vi "test_Set-Get Protocol UDP.vi"(8 "error in (no error)":errorcluster, 11 "TestCase in":refnum<class "Instrument Addon Scripting API Custom Device Unit Tests.lvclass">) -> (0 "error out":errorcluster, 3 "TestCase out":refnum<class "Instrument Addon Scripting API Custom Device Unit Tests.lvclass">)   [LabVIEW 2019, in "Instrument Addon Scripting API Custom Device Unit Tests.lvclass"]
uses:
  Instrument Addon Scripting API Custom Device Unit Tests.lvclass
  Includes/Protocols.lvlibp/UDP/UDP.lvclass
  C:/Users/nitest/Desktop/Git/niveristand-instrument-addon-custom-device/Includes/Protocols.lvlibp/Protocol Parent/Protocol Parent.lvclass
  Includes/Protocols.lvlibp/AK RS-xxx/AK RS-xxx.lvclass
  Instrument Addon Scripting API Custom Device Unit Tests.lvclass/Instrument Addon Scripting API Custom Device Unit Tests.ctl
  Includes/Protocols.lvlibp/UDP/Data Access/Write Local IP Address.vi
  Includes/Protocols.lvlibp/UDP/Data Access/Write Local Port.vi
  Includes/Protocols.lvlibp/UDP/Data Access/Write Target IP Address.vi
  Includes/Protocols.lvlibp/UDP/Data Access/Write Target Port.vi
  Instrument Addon Scripting API Test Assets/Instrument Addon Scripting API Test Assets.lvclass
  <vilib>/addons/_JKI Toolkits/VI Tester/TestCase.llb/TestCase.lvclass
  APIs/Scripting API/Instrument Addon Scripting API.lvlib
  C:/Program Files (x86)/National Instruments/LabVIEW 2019/vi.lib/addons/_JKI Toolkits/VI Tester/TestCase.llb/TestCase.lvclass
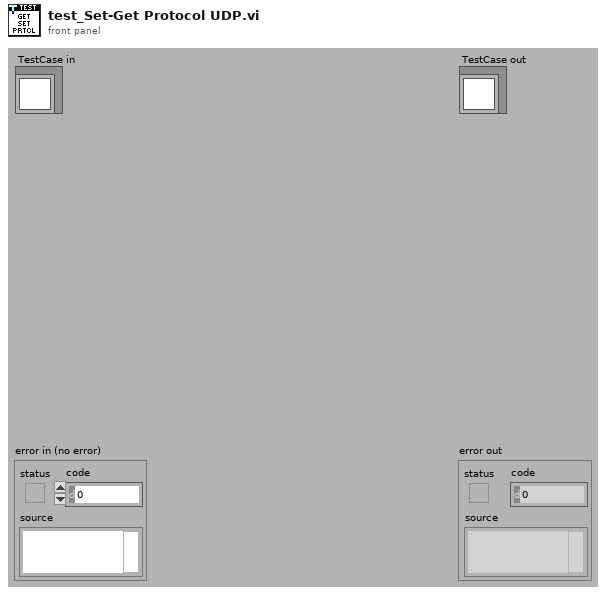
[diagram p1: front panel]
types:
  T1 = typedef "Custom Device API.lvlib/Custom Device Item Ref.ctl" = u64
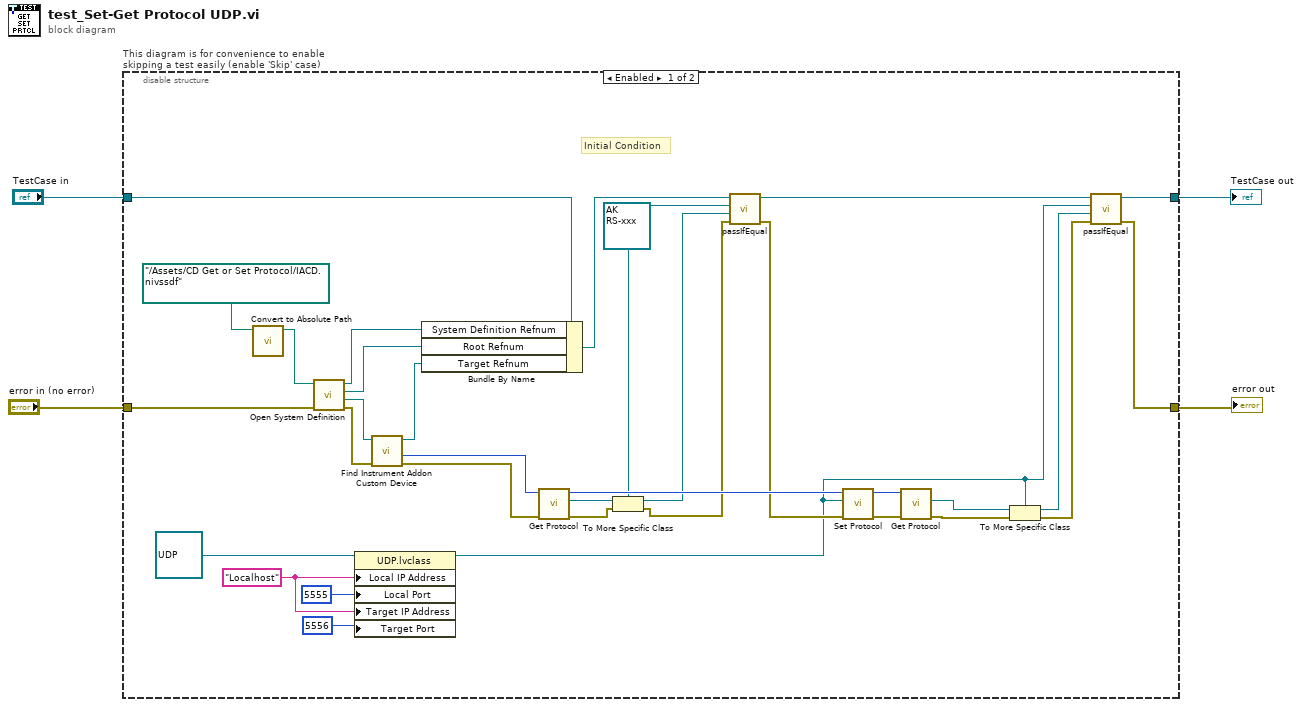
[diagram p0: block diagram]
diagram:
  n1 = disable-structure "This diagram is for convenience to enable skipping a test easily (enable 'Skip' case)" shown="Enabled" {
    disable-tunnel: "TestCase in" -> [w9 w41]
    disable-tunnel: [w27 w39] -> w1
    disable-tunnel: [w25 w40] -> w3
    disable-tunnel: "error in (no error)" -> [w37 w38]
    frame Enabled {
      w11 = refnum<class "AK RS-xxx.lvclass"> refnum ("reference out")
      w21 = "Localhost" ("VISA Resource")
      # "Initial Condition"
      n2 = call "Convert to Absolute Path.vi"("System Definition File"=path "../Assets/CD Get or Set Protocol/IACD.nivssdf" ("SDF file")) -> ("Absolute Path"=w35:path)  [unwired: 10 in]
      n3 = call "Open System Definition.vi"("error in (no error)"=w37, "System Definition File"=w35) -> ("error out"=w34:errorcluster, "Target Refnum"=w33:refnum<k24>, "Root Refnum"=w6:refnum<k24>, "System Definition Refnum"=w7:refnum<k24>)  [unwired: 6 in]
      n4 = property class="UDP.lvclass"(reference=refnum<class "UDP.lvclass"> refnum ("Protocols.lvlibp:UDP.lvclass"), "Local IP Address"=w21, "Local Port"=u16 5555, "Target IP Address"=w21, "Target Port"=u16 5556 ("Local Port")) -> (reference out=w15:refnum<class "UDP.lvclass">)  [unwired: 1 in, 1 out]
      n5 = call "Find Instrument Addon Custom Device.vi"("error in"=w34, "target in"=w33) -> ("error out"=w20:errorcluster, "NodeID"=w19:u64, "target out"=w5:refnum<k24>)  [unwired: 7 in]
      n6 = Bundle By Name(cluster=w9, "System Definition Refnum"=w7, "Root Refnum"=w6, "Target Refnum"=w5) -> (w8:refnum<class "Instrument Addon Scripting API Custom Device Unit Tests.lvclass">)
      n7 = call "Get Protocol.vi"("error in (no error)"=w20, "instrument addon refnum in"=w19) -> ("error out"=w14:errorcluster, "protocol"=w18:refnum<class "Protocol Parent.lvclass">, "instrument addon refnum out"=w17:T1)  [unwired: 7 in]
      n8 = To More Specific Class(target class=w11, reference=w18, error in=w14) -> (specific class reference=w10:refnum<class "AK RS-xxx.lvclass">, error out=w13:errorcluster)
      n9 = call-dynamic "passIfEqual.vi"("error in (no error)"=w13, "y"=w10, "x"=w11, "TestCase in"=w8) -> ("error out"=w16:errorcluster, "TestCase out"=w12:refnum<class "Instrument Addon Scripting API Custom Device Unit Tests.lvclass">)  [unwired: 6 in]
      n10 = call "Set Protocol.vi"("error in (no error)"=w16, "protocol"=w15, "instrument addon refnum in"=w17) -> ("error out"=w31:errorcluster, "instrument addon refnum out"=w32:T1)  [unwired: 7 in]
      n11 = call "Get Protocol.vi"("error in (no error)"=w31, "instrument addon refnum in"=w32) -> ("error out"=w29:errorcluster, "protocol"=w30:refnum<class "Protocol Parent.lvclass">)  [unwired: 7 in, 1 out]
      n12 = To More Specific Class(target class=w15, reference=w30, error in=w29) -> (specific class reference=w26:refnum<class "UDP.lvclass">, error out=w28:errorcluster)
      n13 = call-dynamic "passIfEqual.vi"("error in (no error)"=w28, "y"=w26, "x"=w15, "TestCase in"=w12) -> ("error out"=w25:errorcluster, "TestCase out"=w27:refnum<class "Instrument Addon Scripting API Custom Device Unit Tests.lvclass">)  [unwired: 6 in]
    }
    frame Disabled {
      # "skip test result while test is under development"
      n14 = call <vilib>:"skip.vi"("error in (no error)"=w38, "TestCase in"=w41) -> ("error out"=w40:errorcluster, "TestCase out"=w39:refnum<class "Instrument Addon Scripting API Custom Device Unit Tests.lvclass">)  [unwired: 8 in]
    }
  }
  "error out" <- w3
  "TestCase out" <- w1
